vi "Close.vi"(8 "error in (no error)":errorcluster, 11 "VISA resource name":refnum<visa-resource-name>) -> (0 "error out":errorcluster)   [LabVIEW 2020, in "Control de MaP.lvlib"]
doc: "Close the motors com port communication"
uses:
  Control de MaP.lvlib
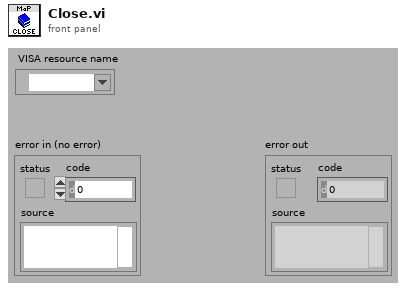
[diagram p1: front panel]
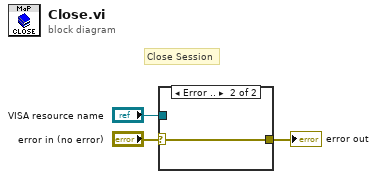
[diagram p0: block diagram]
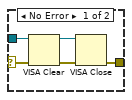
[diagram p2: hidden frame]
diagram:
  # "Close Session"
  n1 = case shown="Error .." "error in (no error)" {
    selector: "error in (no error)" -> [w7 w9]
    tunnel: [w8 w9] -> w3
    tunnel: "VISA resource name" -> [w5 _]
    frame No Error {
      n2 = VISA Clear(VISA resource name=w5, error in (no error)=w7) -> (VISA resource name out=w4:refnum<visa-resource-name>, error out=w6:errorcluster)
      n3 = VISA Close(VISA resource name=w4, error in (no error)=w6) -> (error out=w8:errorcluster)
    }
    frame Error {
    }
  }
  "error out" <- w3
